vi "Read Ini.vi"(0 "Status输入":T1, 5 "错误输入（无错误）":errorcluster) -> (14 "Status输出":T1, 19 "错误输出":errorcluster)   [LabVIEW 2013]
uses:
  Status.ctl
  Step.ctl
  <vilib>/Utility/config.llb/Read Key (String).vi
  <vilib>/Utility/config.llb/NI_LVConfig.lvlib
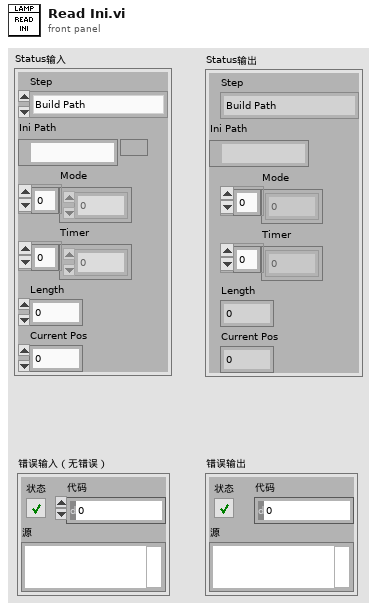
[diagram p1: front panel]
types:
  T1 = typedef "Status.ctl" = cluster{"Step":T2, "Ini Path":path, "Mode":u32[], "Timer":dbl[], "Length":i32, "Current Pos":i32}
  T2 = typedef "Step.ctl" = enum16{"Build Path", "Read Ini", "Run"}
  T3 = typedef "NI_LVConfig.lvlib/Config Data RefNum.ctl" = refnum<k1>
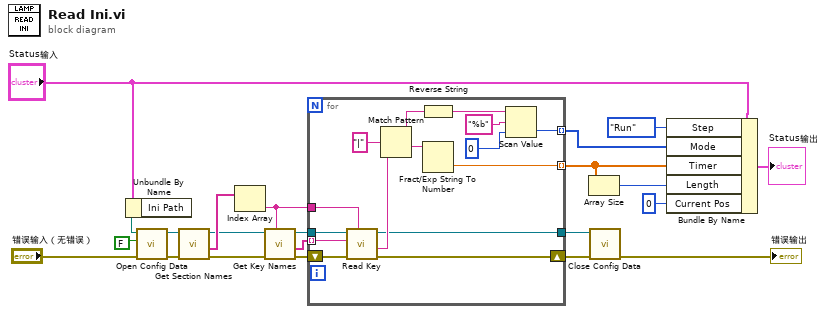
[diagram p0: block diagram]
diagram:
  n1 = Unbundle By Name("Status输入") -> ("Ini Path"=w1:path)
  n2 = call <vilib>:"Open Config Data.vi"("error in (no error)"="错误输入（无错误）", "create file if necessary (T)"=FALSE, "configuration file path"=w1) -> ("error out"=w9:errorcluster, "refnum"=w10:T3)  [unwired: 6 in, 1 out]
  n3 = call <vilib>:"Get Section Names.vi"("error in (no error)"=w9, "refnum"=w10) -> ("error out"=w6:errorcluster, "section names"=w8:string[], "refnum out"=w7:T3)  [unwired: 7 in]
  n4 = Index Array(array=w8) -> (element=w4:string)  [unwired: 1 in]
  n5 = call <vilib>:"Get Key Names.vi"("section"=w4, "error in (no error)"=w6, "refnum"=w7) -> ("error out"=w5:errorcluster, "key names"=w12:string[], "refnum out"=w3:T3)  [unwired: 5 in, 1 out]
  n6 = for {
    shift-right: [w31] -> w14
    shift-left: w5 -> [w37]
    tunnel: w12 -> [w35] mode=indexing
    tunnel: w4 -> [w36]
    tunnel: w3 -> [w34]
    tunnel: [w29] -> w19 mode=indexing
    tunnel: [w26] -> w21 mode=indexing
    tunnel: [w23] -> w16
    n7 = call-poly <vilib>:"Read Key.vi"("section"=w36, "error in (no error)"=w37, "key"=w35, "refnum"=w34) -> ("error out"=w31:errorcluster, "value"=w33:string, "refnum out"=w23:T3)  [unwired: 4 in, 1 out]
    n8 = Match Pattern(string=w33, regular expression="|" ("搜索字符串")) -> (before substring=w25:string, after substring=w27:string)  [unwired: 1 in, 2 out]
    n9 = Reverse String(1:w25) -> (0:w24:string)
    n10 = Fract/Exp String To Number(string=w27) -> (number=w26:dbl)  [unwired: 3 in, 1 out]
    n11 = Scan Value(string=w24, format string="%b" ("格式字符串"), default (0 dbl)=u32 0) -> (value=w29:u32)  [unwired: 1 out]
  }
  n12 = Array Size(array=w21) -> (size(s)=w22:i32)
  n13 = call <vilib>:"Close Config Data.vi"("error in (no error)"=w14, "refnum"=w16) -> ("error out"=→"错误输出":errorcluster)  [unwired: 8 in, 1 out]
  n14 = Bundle By Name(cluster="Status输入", "Step"=Step."Run", "Mode"=w19, "Timer"=w21, "Length"=w22, "Current Pos"=0) -> (→"Status输出":T1)
